vi "1.vi"() -> ()   [LabVIEW 2014]
panel:
  out "XY Graph":cluster{dbl[], dbl[]}(graph)
  in  "Span":dbl
  in  "Start Value":dbl
  in  "Number of Points":dbl
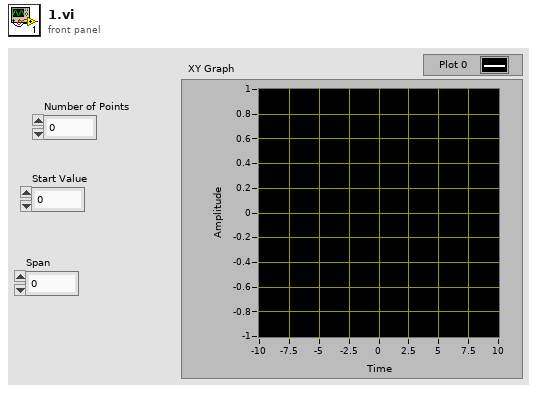
[diagram p1: front panel]
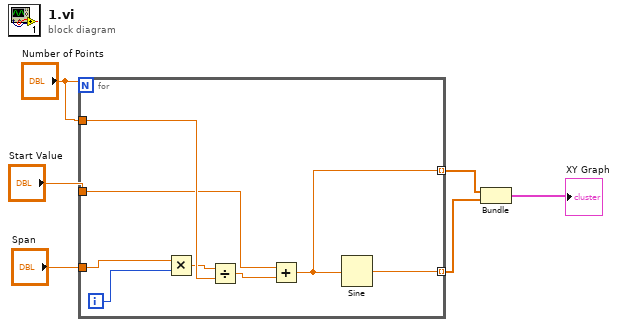
[diagram p0: block diagram]
diagram:
  n1 = for {
    N: "Number of Points" -> [_]
    tunnel: "Start Value" -> [w9]
    tunnel: "Span" -> [w13]
    tunnel: "Number of Points" -> [w12]
    tunnel: [w10] -> w2 mode=indexing
    tunnel: [w7] -> w3 mode=indexing
    i -> [w14]
    n2 = Multiply(x=w13, y=w14) -> (x*y=w11:dbl)
    n3 = Divide(x=w11, y=w12) -> (x/y=w8:dbl)
    n4 = Add(x=w9, y=w8) -> (x+y=w7:dbl)
    n5 = Sine(x=w7) -> (sin(x)=w10:dbl)
  }
  n6 = Bundle(w3, w2) -> (→"XY Graph":cluster{dbl[], dbl[]})  [unwired: 1 in]
